vi "FindChildActorAttributesMap.vi"(11 "Actor":refnum<class "Actor.lvclass">) -> (3 "ChildActorAttributesMap":T1)   [LabVIEW 2020, in "jettl.lvlib"]
uses:
  jettl.lvlib
  Actor/Actor.lvclass
  Msg/Msg.lvclass
  MsgSet.ctl
  Msg.ctl
  PostSetup.ctl
  PreSetup.ctl
  Unified.ctl
  ChildUnifiedMap.ctl
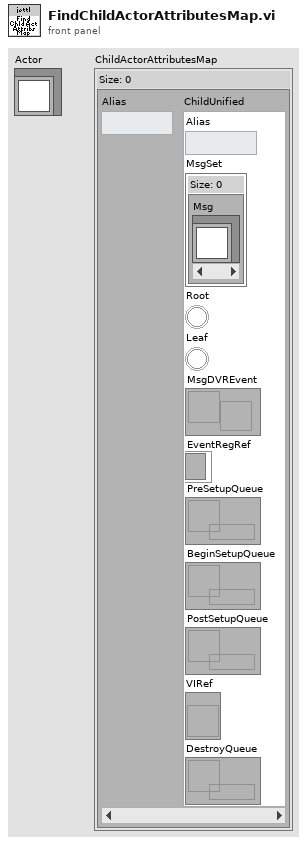
[diagram p1: front panel]
types:
  T1 = typedef "jettl.lvlib/ChildUnifiedMap.ctl" = map{string, T2}
  T2 = typedef "jettl.lvlib/Unified.ctl" = cluster{"Alias":string, "MsgSet":T3, "Root":bool, "Leaf":bool, "MsgDVREvent":refnum<user-event>, "EventRegRef":refnum<event-registration>, "PreSetupQueue":refnum<queue>, "BeginSetupQueue":refnum<queue>, "PostSetupQueue":refnum<queue>, "VIRef":refnum<vi>, "DestroyQueue":refnum<queue>}
  T3 = typedef "jettl.lvlib/MsgSet.ctl" = set{refnum<class "Msg.lvclass">}
  T4 = typedef "jettl.lvlib/Base.ctl" = cluster{"Lifecycle":T5, "SelfUnified":T2, "ParentUnified":T2, "ChildUnifiedMap":T1}
  T5 = typedef "jettl.lvlib/Lifecycle.ctl" = enum16{"Initializing", "SettingUp", "Starting", "Running", "Stopping", "TearingDown", "Terminated"}
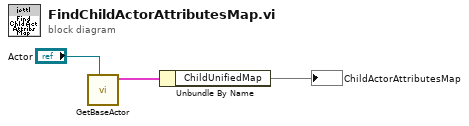
[diagram p0: block diagram]
diagram:
  n1 = call-dynamic "GetBaseActor.vi"("Actor"="Actor") -> ("BaseActor"=w2:T4)  [unwired: 10 in]
  n2 = Unbundle By Name(w2) -> ("ChildUnifiedMap"=→"ChildActorAttributesMap":T1)
